vi "read_basic_log.vi"() -> ()   [LabVIEW 2013]
doc: "Reads the message created by write_basic_log IF the saved variables and the \"read\" variables are the same.\n\nEric Schneider, October 2014"
uses:
  cRIO_Code/Data/TypeDefs/BasicLogReading.ctl
  cRIO_Code/Data/TypeDefs/Sail Set Suggestions.ctl
  cRIO_Code/Data/TypeDefs/Rudder Set Suggestions.ctl
  cRIO_Code/Data/TypeDefs/UTM Location.ctl
panel:
  out "Array of gathered data in a cluster":T1[](array[typedef]) {"SailPositions"."MainSailSuggestion" min=0.0 max=1.0; "SailPositions"."JibSailSuggestion" min=0.0 max=1.0; "RudderPosition" min=-0.95 max=0.95 scale=1.0..-1.0; "BoatLocation"."North" format="%#_10f"; "BoatLocation"."East" format="%#_8f"}
  out "size(s)":i32
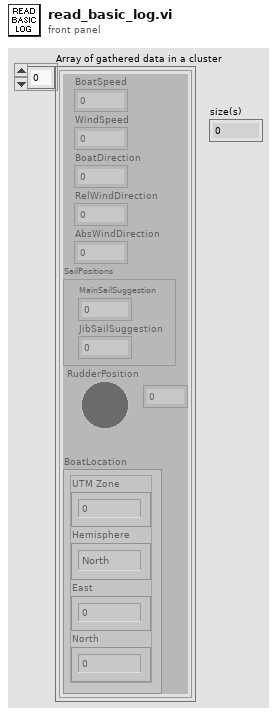
[diagram p1: front panel]
types:
  T1 = typedef "BasicLogReading.ctl" = cluster{"BoatSpeed":dbl, "WindSpeed":dbl, "BoatDirection":dbl, "RelWindDirection":dbl, "AbsWindDirection":dbl, "SailPositions":T2, "RudderPosition":T3, "BoatLocation":T4}
  T2 = typedef "Sail Set Suggestions.ctl" = cluster{"MainSailSuggestion":dbl, "JibSailSuggestion":dbl}
  T3 = typedef "Rudder Set Suggestions.ctl" = dbl
  T4 = typedef "UTM Location.ctl" = cluster{"UTM Zone":dbl, "Hemisphere":enum16{"North", "South"}, "East":dbl, "North":dbl}
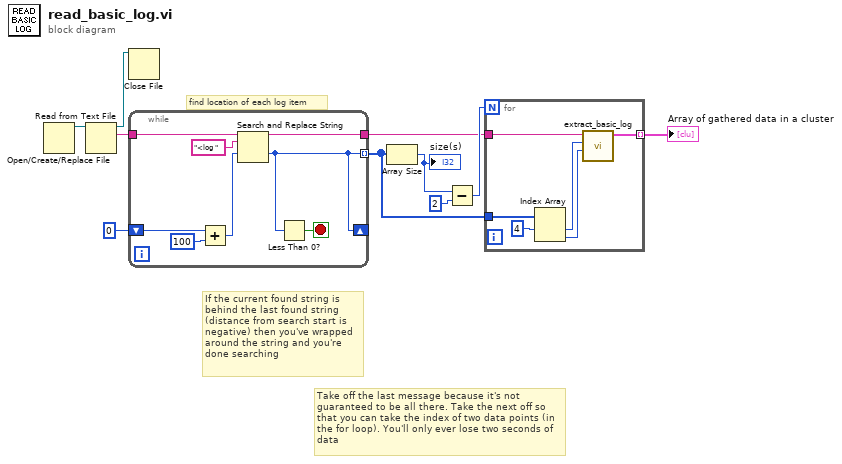
[diagram p0: block diagram]
diagram:
  # "Take off the last message because it's not guaranteed to be all there. Take the next off so that you can take the index of two data points (in the for loop). You'll only ever lose two seconds of data"
  # "If the current found string is behind the last found string (distance from search start is negative) then you've wrapped around the string and you're done searching"
  # "find location of each log item"
  n1 = Open/Create/Replace File() -> (refnum out=w10:refnum<file>)  [unwired: 6 in, 2 out]
  n2 = Read from Text File(file (use dialog)=w10) -> (refnum out=w9:refnum<file>, text=w8:string)  [unwired: 3 in, 2 out]
  n3 = Close File(refnum=w9) -> ()  [unwired: 1 in, 2 out]
  n4 = while {
    tunnel: w8 -> [w18]
    shift-right: [w11] -> _
    shift-left: 0 ("offset past replacement") -> [w15]
    tunnel: [w12] -> w2
    tunnel: [w11] -> w3 mode=indexing
    stop <- w16 stop-if-true
    n5 = Add(x=w15, y=100) -> (x+y=w14:i32)
    n6 = Search and Replace String(input string=w18, search string="<log ", offset=w14) -> (result string=w12:string, offset past replacement=w11:i32)  [unwired: 5 in, 2 out]
    n7 = Less Than 0?(x=w11) -> (x < 0?=w16:bool)
  }
  n8 = Array Size(array=w3) -> (size(s)=w6:i32)
  "size(s)" <- w6
  n9 = Subtract(x=w6, y=2) -> (x-y=w4:i32)
  n10 = for {
    N: w4 -> [_]
    tunnel: w3 -> [w24]
    tunnel: w2 -> [w22]
    tunnel: [w19] -> w1 mode=indexing
    n11 = Index Array(array=w24, index #1=4 ("index")) -> (element #1=w21:i32, element #2=w20:i32)  [unwired: 1 in]
    n12 = call "extract_basic_log.vi"("Next element index"=w20, "Current element index"=w21, "total string"=w22) -> ("Cluster of named data"=w19:T1)  [unwired: 8 in]
  }
  "Array of gathered data in a cluster" <- w1
